vi "Configure.vi"(8 "error in":errorcluster, 10 "name":string, 11 "CRDS in":refnum<class "CRDS.lvclass">) -> (0 "error out":errorcluster, 3 "CRDS out":refnum<class "CRDS.lvclass">)   [LabVIEW 2015, in "CRDS Lib.lvlib" / "CRDS.lvclass"]
doc: "Configure the instrument class. If there is no config file specified, an error"
uses:
  CRDS.lvclass
  Data/Main/CRDS Data.lvclass
  General/Math/Fit Exponential Class/Children/LRS/LRS.lvclass
  General/Math/Fit Exponential Class/Fit Exponential.lvclass/Fit Exponential.ctl
  Instrument/Instrument.lvclass/Instrument.ctl
  Session APIs/File Access/Config Data/Config Data.lvclass/Config Data.ctl
  Data/Cell/CRDS Cell Data.lvclass
  Data/Data.lvclass/Data.ctl
  Data/Cell/CRDS Cell Data.lvclass/CRDS Cell Data.ctl
  Cell/CRDS Cell.lvclass/CRDS Cell.ctl
  Data/Write Data ID.vi
  Data/Cell/Write Ncell.vi
  Data/Cell/Write Write RD_.vi
  Cell/Write ExpFit.vi
  Cell/Write Data.vi
  General/Math/Fit Exponential Class/Write Get A_B.vi
  Instrument/Read Cfg Session.vi
  Session APIs/File Access/Config Data/Accessors/Read Ref.vi
  Instrument/Write Data OK_.vi
  Instrument/Write Data.vi
  Read Cells.vi
  <vilib>/Utility/config.llb/Read Key (I32).vi
  <vilib>/Utility/config.llb/Read Key (Boolean).vi
  Session APIs/File Access/Config Data/Read Array/Read DBL Array.vi
  Session APIs/File Access/Config Data/Read Array/Read String Array.vi
  General/Atmospheric/Atmospheric Constants.vi
  Cell/Write lambda.vi
  Cell/Write optTimeConst.vi
  Data/Main/Write CellData.vi
  Write Cells.vi
  Instrument/Instrument.lvclass
  Cell/CRDS Cell.lvclass
  Session APIs/File Access/Config Data/Config Data.lvclass
  <vilib>/Utility/config.llb/NI_LVConfig.lvlib
  General/Atmospheric/Atmospheric Library.lvlib
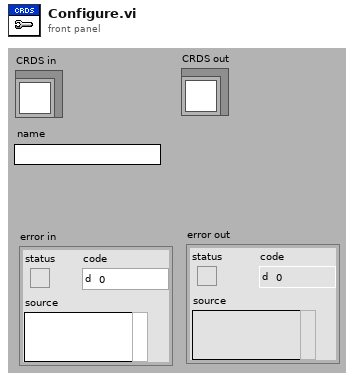
[diagram p1: front panel]
types:
  T1 = typedef "Config Data.lvclass/Config Session.ctl" = refnum<data-value>
  T2 = typedef "NI_LVConfig.lvlib/Config Data RefNum.ctl" = refnum<k1>
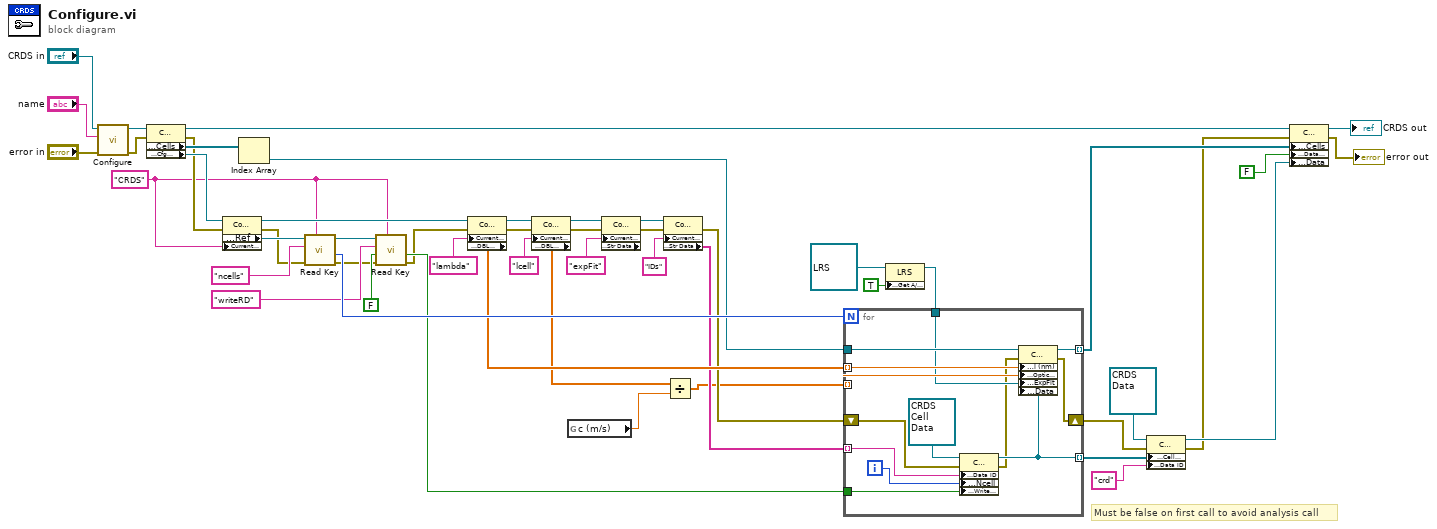
[diagram p0: block diagram]
diagram:
  w12 = "CRDS" ("section")
  # "Must be false on first call to avoid analysis call"
  n1 = call-parent "Configure.vi"("error in"="error in", "name"="name", "Instrument in"="CRDS in") -> ("error out"=w20:errorcluster, "Instrument out"=w48:refnum<class "CRDS.lvclass">)  [unwired: 7 in]
  n2 = property class="CRDS"(reference=w48, error in=w20) -> (reference out=w35:refnum<class "CRDS.lvclass">, error out=w17:errorcluster, "Data Access:Cells"=w18:refnum<class "CRDS Cell.lvclass">[], "Accessors:Cfg Session"=w19:T1)
  n3 = property class="Config Data"(reference=w19, error in=w17, "Current Section"=w12) -> (reference out=w46:T1, error out=w13:errorcluster, "Accessors:Ref"=w14:T2)
  n4 = Index Array(array=w18) -> (element=w38:refnum<class "CRDS Cell.lvclass">)  [unwired: 1 in]
  n5 = call-poly <vilib>:"Read Key.vi"("section"=w12, "error in (no error)"=w13, "key"="ncells", "refnum"=w14) -> ("error out"=w15:errorcluster, "value"=w39:i32, "refnum out"=w16:T2)  [unwired: 4 in, 1 out]
  n6 = call-poly <vilib>:"Read Key.vi"("section"=w12, "error in (no error)"=w15, "default value"=FALSE, "key"="writeRD", "refnum"=w16) -> ("error out"=w11:errorcluster, "value"=w24:bool)  [unwired: 3 in, 2 out]
  n7 = property class="Config Data"(reference=w46, error in=w11, "Current Key"="lambda") -> (reference out=w44:T1, error out=w43:errorcluster, "Read Array Data:DBL Data"=w37:dbl[])
  n8 = property class="Config Data"(reference=w44, error in=w43, "Current Key"="lcell") -> (reference out=w42:T1, error out=w41:errorcluster, "Read Array Data:DBL Data"=w3:dbl[])
  n9 = global read "Atmospheric Constants.vi" "c (m/s)"() -> (w2:dbl)
  n10 = property class="Config Data" props=["Current Key", "Read Array Data:Str Data"](reference=w42, error in=w41, "Current Key"="expFit") -> (reference out=w8:T1, error out=w5:errorcluster)  [unwired: 1 out]
  n11 = property class="Config Data"(reference=w8, error in=w5, "Current Key"="IDs") -> (error out=w4:errorcluster, "Read Array Data:Str Data"=w6:string[])  [unwired: 1 out]
  n12 = Divide(x=w3, y=w2) -> (x/y=w1:dbl[])
  n13 = property class="LRS"(reference=refnum<class "LRS.lvclass"> refnum ("Exponential Fit Lib:LRS"), "Accessors:Get A/B?"=TRUE ("Get A/B?")) -> (reference out=w21:refnum<class "LRS.lvclass">)  [unwired: 1 in, 1 out]
  n14 = for {
    N: w39 -> [_]
    tunnel: w38 -> [w64]
    tunnel: w1 -> [w63] mode=indexing
    tunnel: w37 -> [w62] mode=indexing
    tunnel: [w60] -> w34 mode=indexing
    tunnel: [w57] -> w29 mode=indexing
    tunnel: w21 -> [w59]
    tunnel: w24 -> [w55]
    shift-right: [w61] -> w10
    shift-left: w4 -> [w54]
    tunnel: w6 -> [w52] mode=indexing
    i -> [w56]
    n15 = property class="CRDS Cell"(reference=refnum<class "CRDS Cell Data.lvclass"> refnum ("CRDS Cell"), error in=w54, "Accessors:Data ID"=w52, "Data Access:Ncell"=w56, "Data Access:Write RD_"=w55) -> (reference out=w57:refnum<class "CRDS Cell Data.lvclass">, error out=w53:errorcluster)
    n16 = property class="CRDS Cell"(reference=w64, error in=w53, "Accessors:l (nm)"=w62, "Accessors:Optical Time Constant"=w63, "Accessors:ExpFit"=w59, "Accessors:Data"=w57) -> (reference out=w60:refnum<class "CRDS Cell.lvclass">, error out=w61:errorcluster)
  }
  n17 = property class="CRDS"(reference=refnum<class "CRDS Data.lvclass"> refnum ("CRDS"), error in=w10, "Accessors:Cell Data"=w29, "Accessors:Data ID"="crd" ("Data ID")) -> (reference out=w28:refnum<class "CRDS Data.lvclass">, error out=w9:errorcluster)
  n18 = property class="CRDS"(reference=w35, error in=w9, "Data Access:Cells"=w34, "Accessors:Data OK_"=FALSE ("Data Ready?"), "Accessors:Data"=w28) -> (reference out=→"CRDS out":refnum<class "CRDS.lvclass">, error out=→"error out":errorcluster)
